vi "aft_xmpl_Delay (Array).vi"(8 "error in":errorcluster, 10 "delay":i32, 11 "X":dbl[](array[numeric])) -> (0 "error out":errorcluster, 3 "Delayed X":dbl[](array[numeric]))   [LabVIEW 2019]
uses:
  <vilib>/ptbypt/NI_PtbyPt.lvlib
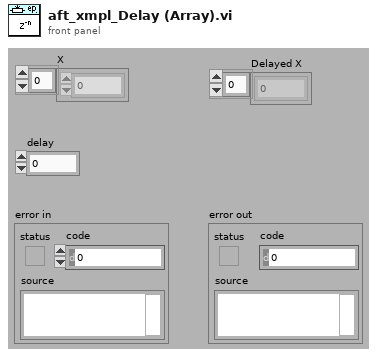
[diagram p1: front panel]
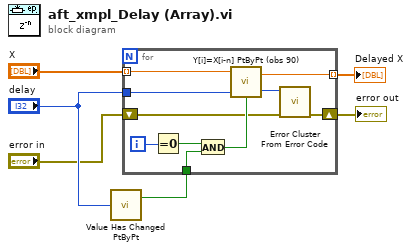
[diagram p0: block diagram]
diagram:
  n1 = call <vilib>:"Value Has Changed PtByPt.vi"("input data point"="delay") -> ("has changed"=w3:bool)  [unwired: 1 in, 1 out]
  n2 = for {
    tunnel: "delay" -> [w16]
    tunnel: "X" -> [w15] mode=indexing
    tunnel: [w14] -> w5 mode=indexing
    tunnel: w3 -> [w11]
    shift-right: [w8] -> w2
    shift-left: "error in" -> [w7]
    i -> [w13]
    n3 = Equal To 0?(x=w13) -> (x = 0?=w12:bool)
    n4 = And(x=w12, y=w11) -> (x .and. y?=w10:bool)
    n5 = call <vilib>:"Y[i]=X[i-n] PtByPt (obs 90).vi"("initialize"=w10, "shifts: n"=w16, "x"=w15) -> ("error"=w9:i32, "shifted x"=w14:dbl)  [unwired: 1 in]
    n6 = call <vilib>:"Error Cluster From Error Code.vi"("error in (no error)"=w7, "error code (0)"=w9) -> ("error out"=w8:errorcluster)  [unwired: 1 in, 6 out]
  }
  "Delayed X" <- w5
  "error out" <- w2
